vi "StepLoadUI.vi"(11 "base path":path) -> (2 "Cancelled?":bool, 3 "Step":T2)   [LabVIEW 2016]
uses:
  <vilib>/Utility/file.llb/Read Delimited Spreadsheet (string).vi
panel:
  in  "Arguments":T1
  in  "Cancel Button":bool
  in  "Add Button":bool
  in  "StepNumber":i32
  in  "StepFiles":i32(listbox)=7
  out "StepData":string[](array[string])=["//_MACRO_STEP-1", "macro:OpenLoopDrive,TRUE,1,0,3,,,,,;"]
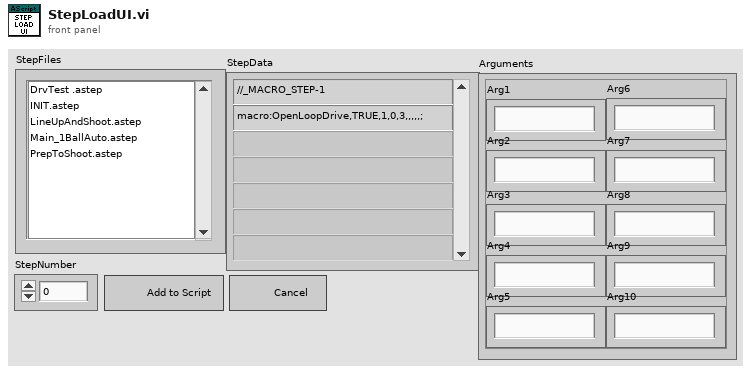
[diagram p1: front panel]
types:
  T1 = cluster{"Arg1":string, "Arg2":string, "Arg3":string, "Arg4":string, "Arg5":string, "Arg6":string, "Arg7":string, "Arg8":string, "Arg9":string, "Arg10":string}
  T2 = cluster{"Number":i32, "Name":string, "Commands":string[], "WaitForExecution":bool}
  T3 = cluster{"Number":i32, "Name":string, "Commands":string[], "WaitForExecution":bool}[]
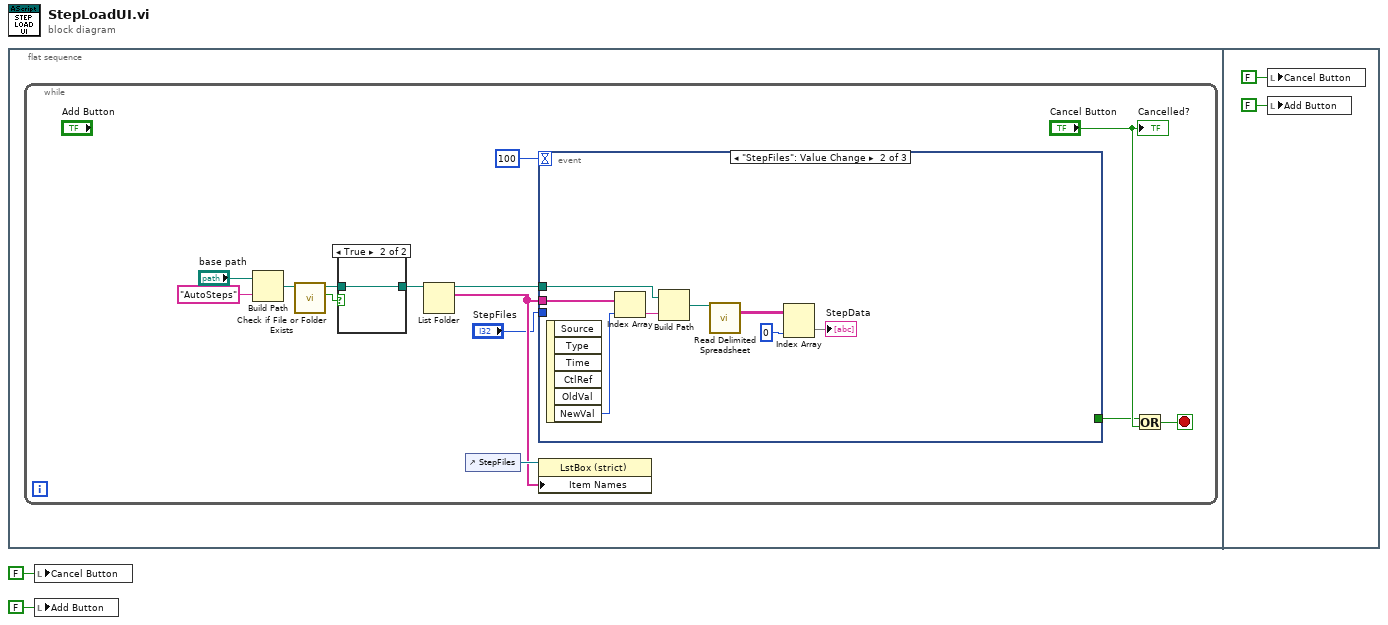
[diagram p0: block diagram]
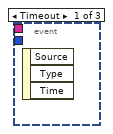
[diagram p2: hidden frame]
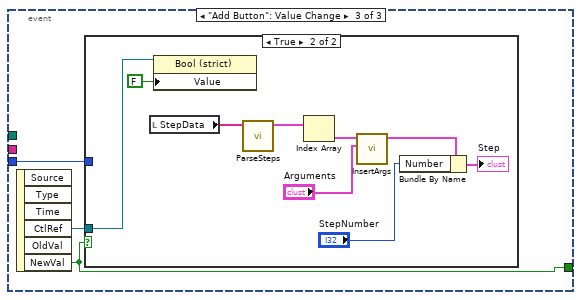
[diagram p3: hidden frame]
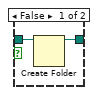
[diagram p5: hidden frame]
diagram:
  n1 = flat-sequence {
    frame #0 {
      n2 = while {
        stop <- w4 stop-if-true
        n3 = Build Path(base path="base path", name or relative path="AutoSteps") -> (appended path=w7:path)
        n4 = call <vilib>:"Check if File or Folder Exists.vi"("path"=w7) -> ("file or folder exists?"=w16:bool, "dup path"=w15:path)  [unwired: 8 in, 1 out]
        n5 = case shown="True" w16 {
          tunnel: w15 -> [w38 w39]
          tunnel: [w37 w39] -> w14
          frame False {
            n6 = Create Folder(path (use dialog)=w38) -> (created path=w37:path)  [unwired: 2 in, 2 out]
          }
          frame True {
          }
        }
        n7 = List Folder(path=w14) -> (path out=w10:path, filenames=w12:string[])  [unwired: 3 in, 2 out]
        n8 = control-ref of="StepFiles"() -> (w13:refnum<vi>)
        n9 = event shown="[1] \"StepFiles\": Value Change" {
          selector: _ -> [_ _ _]
          dyn-events: _ -> [_ _ _]
          timeout: 100 -> [_ _ _]
          tunnel: w12 -> [_ w23 _]
          tunnel: w10 -> [_ w21 _]
          tunnel: "StepFiles" -> [_ _ w27]
          tunnel: [_ _ w25] -> w5
          event Timeout {
            n10 = event-data() -> ()  [unwired: 1 in, 3 out]
          }
          event "StepFiles": Value Change {
            n11 = event-data() -> ("NewVal"=w24:i32)  [unwired: 1 in, 5 out]
            n12 = Index Array(array=w23, index=w24) -> (element=w22:string)
            n13 = Build Path(base path=w21, name or relative path=w22) -> (appended path=w18:path)
            n14 = call-poly <vilib>:"Read Delimited Spreadsheet.vi"("file path (dialog if empty)"=w18) -> ("all rows"=w19:string[][])  [unwired: 9 in, 5 out]
            n15 = Index Array(array=w19, index (col)=0 ("disabled index (col)")) -> (element=→"StepData":string[])  [unwired: 1 in]
          }
          event "Add Button": Value Change {
            n16 = event-data() -> ("CtlRef"=w26:refnum<vi>, "NewVal"=w25:bool)  [unwired: 1 in, 4 out]
            n17 = case shown="True" w25 {
              tunnel: w27 -> [_ _]
              tunnel: w26 -> [_ w32]
              frame False {
              }
              frame True {
                n18 = local read "StepData"() -> (w36:string[])
                n19 = property class="Bool (strict)"(reference=w32, "Value"=FALSE) -> ()  [unwired: 1 in, 2 out]
                n20 = call "ParseSteps.vi"("AscriptLines"=w36) -> ("Steps"=w35:T3)  [unwired: 10 in]
                n21 = Index Array(array=w35) -> (element=w30:T2)  [unwired: 1 in]
                n22 = call "InsertArgs.vi"("Arguments"="Arguments", "StepIn"=w30) -> ("StepOut"=w29:T2)  [unwired: 9 in]
                n23 = Bundle By Name(cluster=w29, "Number"="StepNumber") -> (→"Step":T2)
              }
            }
          }
        }
        n24 = property on="Property Node" class="LstBox (strict)"(reference=w13, "Item Names"=w12) -> ()  [unwired: 1 in, 2 out]
        n25 = Or(x=w5, y="Cancel Button") -> (x .or. y?=w4:bool)
        "Cancelled?" <- "Cancel Button"
      }
    }
    frame #1 {
      n26 = local write "Cancel Button"(FALSE ("Cancel Button")) -> ()
      n27 = local write "Add Button"(FALSE ("Cancel Button")) -> ()
    }
  }
  n28 = local write "Cancel Button"(FALSE ("Cancel Button")) -> ()
  n29 = local write "Add Button"(FALSE ("Cancel Button")) -> ()
